vi "Get FPGA Reference.vi"(8 "Error In":errorcluster, 11 "Display In":refnum<class "Neopixel - Host.lvclass">) -> (0 "Error Out":errorcluster, 2 "FPGA VI Reference":T1, 3 "Display Out":refnum<class "Neopixel - Host.lvclass">)   [LabVIEW 2021, in "Neopixel - Host.lvclass"]
uses:
  Neopixel - Host.lvclass
  Public/Controls/FPGA Reference.ctl
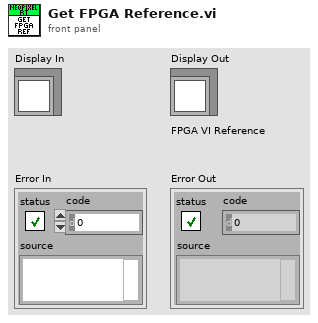
[diagram p1: front panel]
types:
  T1 = typedef "Neopixel - Host.lvclass/FPGA Reference.ctl" = refnum<k20>
  T2 = typedef "Neopixel - RT.lvclass/Data.ctl" = cluster{"FPGA VI Reference":T3, "RGB Gains":T4}
  T3 = typedef "Neopixel - RT.lvclass/FPGA Reference.ctl" = refnum<k20>
  T4 = typedef "Neopixel - RT.lvclass/RGB Gains.ctl" = cluster{"Red":sgl, "Green":sgl, "Blue":sgl}
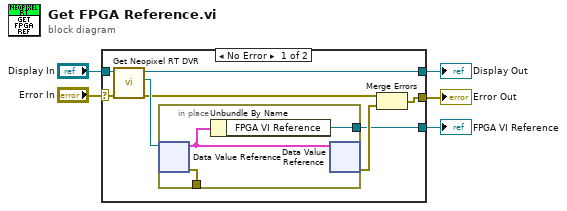
[diagram p0: block diagram]
diagram:
  n1 = case shown="No Error" "Error In" {
    selector: "Error In" -> [w9 w17]
    tunnel: [w11 w17] -> w2
    tunnel: [w8 w18] -> w3
    tunnel: "Display In" -> [w10 w18]
    tunnel: [w12 _] -> w1
    frame No Error {
      n2 = call "Get Neopixel RT DVR.vi"("Error In"=w9, "Display In"=w10) -> ("Error Out"=w6:errorcluster, "DVR"=w7:refnum<data-value>, "Display Out"=w8:refnum<class "Neopixel - Host.lvclass">)  [unwired: 7 in]
      n3 = in-place {
        in-place-border: [w14] -> w12
        in-place-border: [w16] -> _
        n4 = in-place-dvr #1(w7) -> (w15:T2, w16:errorcluster)
        n5 = Unbundle By Name(w15) -> ("FPGA VI Reference"=w14:T3)
        n6 = in-place-dvr #1(w15) -> (w13:errorcluster)  [unwired: 1 out]
      }
      n7 = Merge Errors(w6, w13) -> (w11:errorcluster)
    }
    frame Error {
    }
  }
  "Error Out" <- w2
  "Display Out" <- w3
  "FPGA VI Reference" <- w1
